vi "黑白棋.vi"() -> ()   [LabVIEW 2021]
panel:
  out "落子者計算":i32
  out "現落子者":bool
  in  "重啟棋局":bool
  in  "Boolean 25":bool
  in  "Boolean 24":bool
  in  "Boolean 23":bool
  in  "Boolean 22":bool
  in  "Boolean 21":bool
  in  "Boolean 20":bool
  in  "Boolean 19":bool
  in  "Boolean 18":bool
  in  "Boolean 17":bool
  in  "Boolean 16":bool
  in  "Boolean 15":bool
  in  "Boolean 14":bool
  in  "Boolean 13":bool
  in  "Boolean 12":bool
  in  "Boolean 11":bool
  in  "Boolean 10":bool
  in  "Boolean 9":bool
  in  "Boolean 8":bool
  in  "Boolean 7":bool
  in  "Boolean 6":bool
  in  "Boolean 5":bool
  in  "Boolean 4":bool
  in  "Boolean 3":bool
  in  "Boolean 2":bool
  in  "Boolean":bool
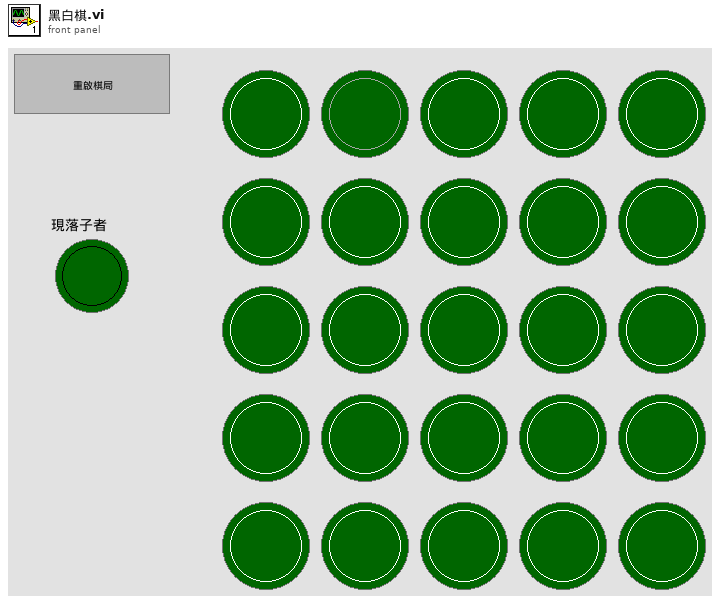
[diagram p1: front panel]
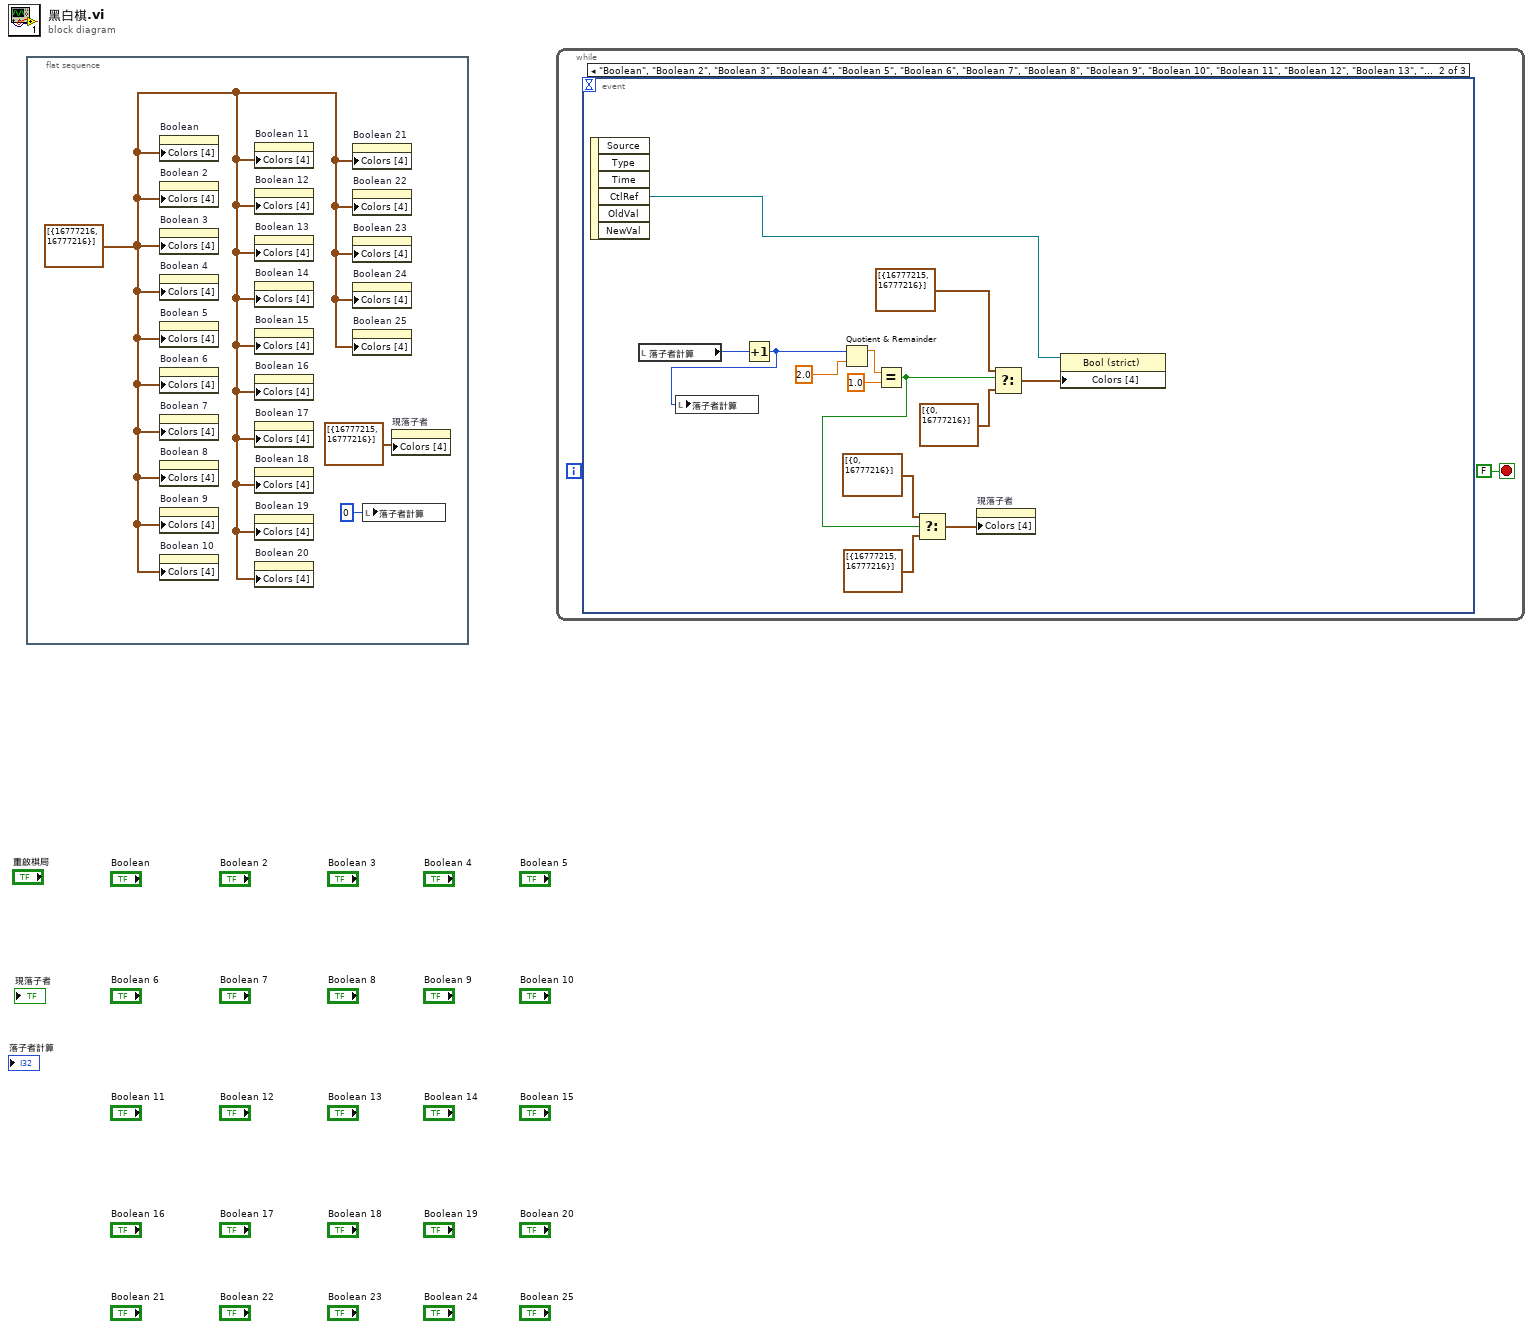
[diagram p0: block diagram]
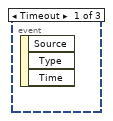
[diagram p2: hidden frame]
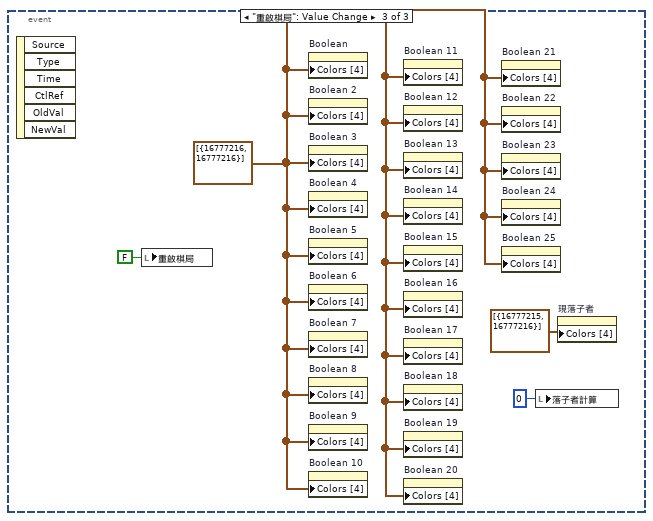
[diagram p3: hidden frame]
diagram:
  n1 = flat-sequence {
    frame #0 {
      w3 = cluster{u32, u32}[] [{16777216, 16777216}] ("Colors [4]")
      n2 = property on="Boolean" class="Bool (strict)"("Colors [4]"=w3) -> ()  [unwired: 2 in, 2 out]
      n3 = property on="Boolean 2" class="Bool (strict)"("Colors [4]"=w3) -> ()  [unwired: 2 in, 2 out]
      n4 = property on="Boolean 3" class="Bool (strict)"("Colors [4]"=w3) -> ()  [unwired: 2 in, 2 out]
      n5 = property on="Boolean 4" class="Bool (strict)"("Colors [4]"=w3) -> ()  [unwired: 2 in, 2 out]
      n6 = property on="Boolean 5" class="Bool (strict)"("Colors [4]"=w3) -> ()  [unwired: 2 in, 2 out]
      n7 = property on="Boolean 6" class="Bool (strict)"("Colors [4]"=w3) -> ()  [unwired: 2 in, 2 out]
      n8 = property on="Boolean 7" class="Bool (strict)"("Colors [4]"=w3) -> ()  [unwired: 2 in, 2 out]
      n9 = property on="Boolean 8" class="Bool (strict)"("Colors [4]"=w3) -> ()  [unwired: 2 in, 2 out]
      n10 = property on="Boolean 9" class="Bool (strict)"("Colors [4]"=w3) -> ()  [unwired: 2 in, 2 out]
      n11 = property on="Boolean 10" class="Bool (strict)"("Colors [4]"=w3) -> ()  [unwired: 2 in, 2 out]
      n12 = property on="Boolean 11" class="Bool (strict)"("Colors [4]"=w3) -> ()  [unwired: 2 in, 2 out]
      n13 = property on="Boolean 12" class="Bool (strict)"("Colors [4]"=w3) -> ()  [unwired: 2 in, 2 out]
      n14 = property on="Boolean 13" class="Bool (strict)"("Colors [4]"=w3) -> ()  [unwired: 2 in, 2 out]
      n15 = property on="Boolean 14" class="Bool (strict)"("Colors [4]"=w3) -> ()  [unwired: 2 in, 2 out]
      n16 = property on="Boolean 15" class="Bool (strict)"("Colors [4]"=w3) -> ()  [unwired: 2 in, 2 out]
      n17 = property on="Boolean 16" class="Bool (strict)"("Colors [4]"=w3) -> ()  [unwired: 2 in, 2 out]
      n18 = property on="Boolean 17" class="Bool (strict)"("Colors [4]"=w3) -> ()  [unwired: 2 in, 2 out]
      n19 = property on="Boolean 18" class="Bool (strict)"("Colors [4]"=w3) -> ()  [unwired: 2 in, 2 out]
      n20 = property on="Boolean 19" class="Bool (strict)"("Colors [4]"=w3) -> ()  [unwired: 2 in, 2 out]
      n21 = property on="Boolean 20" class="Bool (strict)"("Colors [4]"=w3) -> ()  [unwired: 2 in, 2 out]
      n22 = property on="Boolean 21" class="Bool (strict)"("Colors [4]"=w3) -> ()  [unwired: 2 in, 2 out]
      n23 = property on="Boolean 22" class="Bool (strict)"("Colors [4]"=w3) -> ()  [unwired: 2 in, 2 out]
      n24 = property on="Boolean 23" class="Bool (strict)"("Colors [4]"=w3) -> ()  [unwired: 2 in, 2 out]
      n25 = property on="Boolean 24" class="Bool (strict)"("Colors [4]"=w3) -> ()  [unwired: 2 in, 2 out]
      n26 = property on="Boolean 25" class="Bool (strict)"("Colors [4]"=w3) -> ()  [unwired: 2 in, 2 out]
      n27 = local write "落子者計算"(0 ("落子者計算")) -> ()
      n28 = property on="現落子者" class="Bool (strict)"("Colors [4]"=cluster{u32, u32}[] [{16777215, 16777216}]) -> ()  [unwired: 2 in, 2 out]
    }
  }
  n29 = while {
    stop <- FALSE stop-if-true
    n30 = event shown="[1] \"Boolean\", \"Boolean 2\", \"Boolean 3\", \"Boolean 4\", \"Boolean 5\", \"Boolean 6\", \"Boolean 7\", \"Boolean 8\", \"Boolean 9\", \"Boolean 10\", \"Boolean 11\", \"Boolean 12\", \"Boolean 13\", \"Boolean 14\", \"Boolean 15\", \"Boolean 16\", \"Boolean 17\", \"Boolean 18\", \"Boolean 19\", \"Boolean 20\", \"Boolean 21\", \"Boolean 22\", \"Boolean 23\", \"Boolean 24\", \"Boolean 25\": Value Change" {
      selector: _ -> [_ _ _]
      dyn-events: _ -> [_ _ _]
      timeout: _ -> [_ _ _]
      event Timeout {
        n31 = event-data() -> ()  [unwired: 1 in, 3 out]
      }
      event "Boolean", "Boolean 2", "Boolean 3", "Boolean 4", "Boolean 5", "Boolean 6", "Boolean 7", "Boolean 8", "Boolean 9", "Boolean 10", "Boolean 11", "Boolean 12", "Boolean 13", "Boolean 14", "Boolean 15", "Boolean 16", "Boolean 17", "Boolean 18", "Boolean 19", "Boolean 20", "Boolean 21", "Boolean 22", "Boolean 23", "Boolean 24", "Boolean 25": Value Change {
        n32 = event-data() -> ("CtlRef"=w12:refnum<vi>)  [unwired: 1 in, 5 out]
        n33 = local read "落子者計算"() -> (w6:i32)
        n34 = Increment(x=w6) -> (x+1=w5:i32)
        n35 = local write "落子者計算"(w5) -> ()
        n36 = Quotient & Remainder(x=w5, y=2.0) -> (x-y*floor(x/y)=w11:dbl)  [unwired: 1 out]
        n37 = Equal?(x=w11, y=1.0) -> (x = y?=w7:bool)
        n38 = Select(t=cluster{u32, u32}[] [{0, 16777216}] ("Colors [4]"), s=w7, f=cluster{u32, u32}[] [{16777215, 16777216}] ("Colors [4]")) -> (s? t:f=w8:cluster{u32, u32}[])
        n39 = property on="現落子者" class="Bool (strict)"("Colors [4]"=w8) -> ()  [unwired: 2 in, 2 out]
        n40 = Select(t=cluster{u32, u32}[] [{16777215, 16777216}] ("Colors [4]"), s=w7, f=cluster{u32, u32}[] [{0, 16777216}] ("Colors [4]")) -> (s? t:f=w13:cluster{u32, u32}[])
        n41 = property class="Bool (strict)"(reference=w12, "Colors [4]"=w13) -> ()  [unwired: 1 in, 2 out]
      }
      event "重啟棋局": Value Change {
        w21 = cluster{u32, u32}[] [{16777216, 16777216}] ("Colors [4]")
        n42 = event-data() -> ()  [unwired: 1 in, 6 out]
        n43 = local write "重啟棋局"(FALSE ("重啟棋局")) -> ()
        n44 = property on="Boolean" class="Bool (strict)"("Colors [4]"=w21) -> ()  [unwired: 2 in, 2 out]
        n45 = property on="Boolean 2" class="Bool (strict)"("Colors [4]"=w21) -> ()  [unwired: 2 in, 2 out]
        n46 = property on="Boolean 3" class="Bool (strict)"("Colors [4]"=w21) -> ()  [unwired: 2 in, 2 out]
        n47 = property on="Boolean 4" class="Bool (strict)"("Colors [4]"=w21) -> ()  [unwired: 2 in, 2 out]
        n48 = property on="Boolean 5" class="Bool (strict)"("Colors [4]"=w21) -> ()  [unwired: 2 in, 2 out]
        n49 = property on="Boolean 6" class="Bool (strict)"("Colors [4]"=w21) -> ()  [unwired: 2 in, 2 out]
        n50 = property on="Boolean 7" class="Bool (strict)"("Colors [4]"=w21) -> ()  [unwired: 2 in, 2 out]
        n51 = property on="Boolean 8" class="Bool (strict)"("Colors [4]"=w21) -> ()  [unwired: 2 in, 2 out]
        n52 = property on="Boolean 9" class="Bool (strict)"("Colors [4]"=w21) -> ()  [unwired: 2 in, 2 out]
        n53 = property on="Boolean 10" class="Bool (strict)"("Colors [4]"=w21) -> ()  [unwired: 2 in, 2 out]
        n54 = property on="Boolean 11" class="Bool (strict)"("Colors [4]"=w21) -> ()  [unwired: 2 in, 2 out]
        n55 = property on="Boolean 12" class="Bool (strict)"("Colors [4]"=w21) -> ()  [unwired: 2 in, 2 out]
        n56 = property on="Boolean 13" class="Bool (strict)"("Colors [4]"=w21) -> ()  [unwired: 2 in, 2 out]
        n57 = property on="Boolean 14" class="Bool (strict)"("Colors [4]"=w21) -> ()  [unwired: 2 in, 2 out]
        n58 = property on="Boolean 15" class="Bool (strict)"("Colors [4]"=w21) -> ()  [unwired: 2 in, 2 out]
        n59 = property on="Boolean 16" class="Bool (strict)"("Colors [4]"=w21) -> ()  [unwired: 2 in, 2 out]
        n60 = property on="Boolean 17" class="Bool (strict)"("Colors [4]"=w21) -> ()  [unwired: 2 in, 2 out]
        n61 = property on="Boolean 18" class="Bool (strict)"("Colors [4]"=w21) -> ()  [unwired: 2 in, 2 out]
        n62 = property on="Boolean 19" class="Bool (strict)"("Colors [4]"=w21) -> ()  [unwired: 2 in, 2 out]
        n63 = property on="Boolean 20" class="Bool (strict)"("Colors [4]"=w21) -> ()  [unwired: 2 in, 2 out]
        n64 = property on="Boolean 21" class="Bool (strict)"("Colors [4]"=w21) -> ()  [unwired: 2 in, 2 out]
        n65 = property on="Boolean 22" class="Bool (strict)"("Colors [4]"=w21) -> ()  [unwired: 2 in, 2 out]
        n66 = property on="Boolean 23" class="Bool (strict)"("Colors [4]"=w21) -> ()  [unwired: 2 in, 2 out]
        n67 = property on="Boolean 24" class="Bool (strict)"("Colors [4]"=w21) -> ()  [unwired: 2 in, 2 out]
        n68 = property on="Boolean 25" class="Bool (strict)"("Colors [4]"=w21) -> ()  [unwired: 2 in, 2 out]
        n69 = local write "落子者計算"(0 ("落子者計算")) -> ()
        n70 = property on="現落子者" class="Bool (strict)"("Colors [4]"=cluster{u32, u32}[] [{16777215, 16777216}]) -> ()  [unwired: 2 in, 2 out]
      }
    }
  }
